vi "Track Open.vi"() -> ()   [LabVIEW 2011]
uses:
  Robot Global Data.vi
  System Set Points and States.vi
panel:
  in  "time delay":dbl
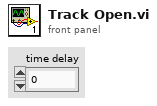
[diagram p1: front panel]
types:
  T1 = typedef "WPI_RobotDriveDevRef.ctl" = cluster{"DevStatus":errorcluster, "Motors[]":T2[], "Square Inputs":bool, "Max Output":dbl, "Isochronous":bool}
  T2 = typedef "WPI_MotorControlDeviceRef.ctl" = cluster{"DeviceStatus":errorcluster, "Type":enum16{"PWM", "CAN"}, "PWM":cluster{"Digital Module":T3, "PWM Channel":T4, "DeadBand":T5}, "CAN":cluster{"Device Number":u8, "Control Mode":T6, "Semaphore":T7, "Max Vout":dbl}, "Invert":bool, "TransformRef":T8, "InvTransformRef":T8}
  T3 = typedef "FPGA_TypedefDigitalModule.ctl" = enum16{"Digital Module 1", "Digital Module 2"}
  T4 = typedef "FPGA_DIOPWMChannel.ctl" = enum8{"PWM 1", "PWM 2", "PWM 3", "PWM 4", "PWM 5", "PWM 6", "PWM 7", "PWM 8", "PWM 9", "PWM 10", "Invalid"}
  T5 = typedef "WPI_PWMDeadband.ctl" = cluster{"Name":string, "maxPositivePwm":i32, "minPositivePwm":i32, "centerPwm":i32, "maxNegativePwm":i32, "minNegativePwm":i32, "angularRange":u16}
  T6 = typedef "WPI_CANJaguar_ControlMode.ctl" = enum8{"Percent VBus", "Current", "Speed", "Position", "Voltage"}
  T7 = typedef "Semaphore RefNum" = refnum<k1>
  T8 = typedef "WPI_PWMTransform_ConPane.ctl" = refnum<vi>
  T9 = typedef "WPI_GyroDevRef.ctl" = cluster{"DevStatus":errorcluster, "Analog Module":T10, "Analog Channel":T11, "Offset":dbl, "Gain (VoltsPerDegree/Second)":dbl}
  T10 = typedef "FPGA_TypedefAnalogModule.ctl" = enum16{"Analog Module 1", "Analog Module 2"}
  T11 = typedef "FPGA_AIChannel.ctl" = enum8{"AI 1", "AI 2", "AI 3", "AI 4", "AI 5", "AI 6", "AI 7", "AI 8", "Invalid"}
  T12 = cluster{"Position":cluster{"X":dbl, "Y":dbl}, "Distance (ft)":dbl}[]
  T13 = cluster{"Position":cluster{"X":dbl, "Y":dbl}, "Distance (ft)":dbl}
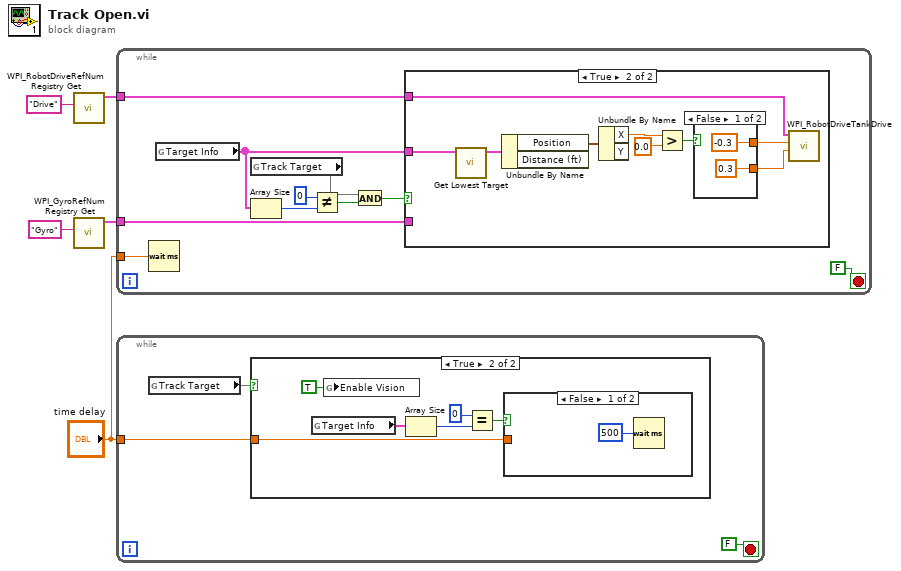
[diagram p0: block diagram]
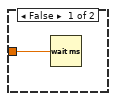
[diagram p2: hidden frame]
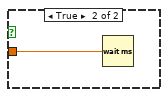
[diagram p3: hidden frame]
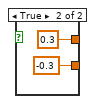
[diagram p5: hidden frame]
diagram:
  n1 = call <vilib>:"WPI_RobotDriveRefNum Registry Get.vi"("refnum name"="Drive") -> ("RobotDriveDevRef"=w2:T1)  [unwired: 9 in, 1 out]
  n2 = call <vilib>:"WPI_GyroRefNum Registry Get.vi"("refnum name"="Gyro") -> ("GyroDevRef"=w4:T9)  [unwired: 9 in, 1 out]
  n3 = while {
    tunnel: w4 -> [w15]
    tunnel: "time delay" -> [w12]
    tunnel: w2 -> [w14]
    stop <- FALSE stop-if-true
    n4 = Wait (ms)(milliseconds to wait=w12) -> ()  [unwired: 1 out]
    n5 = global read "Robot Global Data.vi" "Target Info"() -> (w6:T12)
    n6 = global read "System Set Points and States.vi" "Track Target"() -> (w9)
    n7 = Array Size(array=w6) -> (size(s)=w8:i32)
    n8 = Not Equal?(x=0, y=w8) -> (x != y?=w10:bool)
    n9 = And(x=w9, y=w10) -> (x .and. y?=w11:bool)
    n10 = case shown="True" w11 {
      tunnel: w14 -> [_ w24]
      tunnel: w15 -> [_ _]
      tunnel: w6 -> [_ w23]
      frame False {
      }
      frame True {
        n11 = call "Get Lowest Target.vi"("Target Info"=w23) -> ("Cluster"=w22:T13)  [unwired: 10 in]
        n12 = Unbundle By Name(w22) -> ("Position"=w21:cluster{"X":dbl, "Y":dbl})  [unwired: 1 out]
        n13 = Unbundle By Name(w21) -> ("X"=w20:dbl)  [unwired: 1 out]
        n14 = Greater?(x=w20, y=0.0) -> (0:w18:bool)
        n15 = case shown="False" w18 {
          tunnel: [-0.3 0.3] -> w17
          tunnel: [0.3 -0.3] -> w16
          frame False {
          }
          frame True {
          }
        }
        n16 = call <vilib>:"WPI_RobotDriveTankDrive.vi"("Right axis value"=w16, "Left axis value"=w17, "RobotDriveDevRef"=w24) -> ()  [unwired: 7 in, 2 out]
      }
    }
  }
  n17 = while {
    tunnel: "time delay" -> [w30]
    stop <- FALSE stop-if-true
    n18 = global read "System Set Points and States.vi" "Track Target"() -> (w31)
    n19 = case shown="True" w31 {
      tunnel: w30 -> [w32 w33]
      frame False {
        n20 = Wait (ms)(milliseconds to wait=w32) -> ()  [unwired: 1 out]
      }
      frame True {
        n21 = global read "Robot Global Data.vi" "Target Info"() -> (w38:T12)
        n22 = global write "Robot Global Data.vi" "Enable Vision"(TRUE) -> ()
        n23 = Array Size(array=w38) -> (size(s)=w36:i32)
        n24 = Equal?(x=0, y=w36) -> (x = y?=w37:bool)
        n25 = case shown="False" w37 {
          tunnel: w33 -> [_ w40]
          frame False {
            n26 = Wait (ms)(milliseconds to wait=500) -> ()  [unwired: 1 out]
          }
          frame True {
            n27 = Wait (ms)(milliseconds to wait=w40) -> ()  [unwired: 1 out]
          }
        }
      }
    }
  }
